vi "HC-Sr501.vi"() -> ()   [LabVIEW 2021]
uses:
  <vilib>/MakerHub/LINX/Public/Peripherals/Digital/Digital Read 1 Chan.vi
  <vilib>/MakerHub/LINX/Public/Peripherals/Digital/Digital Read N Chans.vi
  <vilib>/MakerHub/LINX/Private/Local IO/LinxDigitalRead.vi
  <vilib>/MakerHub/LINX/Public/Utilities/Check Channel.vi
  <vilib>/MakerHub/LINX/Public/Utilities/Open Serial.vi
  <vilib>/MakerHub/LINX/Public/Sensors/Motion/Servo/Servo Open One Channel.vi
  <vilib>/MakerHub/LINX/Private/Utilties/Generate Error.vi
  <vilib>/MakerHub/LINX/Public/Sensors/Motion/Servo/Servo Set Pulse Width One Channel.vi
  <vilib>/MakerHub/LINX/Public/Sensors/Motion/Servo/Servo Close One Channel.vi
  <vilib>/MakerHub/LINX/LMH-LINX.lvlib
  <vilib>/MakerHub/LINX/Public/Sensors/Motion/Servo/Servo.lvlib
panel:
  out "DOOR":bool
  in  "stop":bool
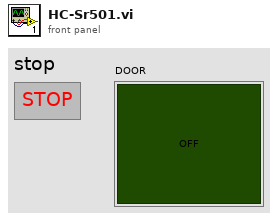
[diagram p1: front panel]
types:
  T1 = typedef "LMH-LINX.lvlib/LINX Ref.ctl" = cluster{"IO":T2, "Interface":T3, "LINX Device Config":T4}
  T2 = typedef "LMH-LINX.lvlib/Platform.ctl" = enum16{"Remote", "Local"}
  T3 = typedef "LMH-LINX.lvlib/Interface.ctl" = enum16{"Serial", "TCP"}
  T4 = typedef "LMH-LINX.lvlib/Device.lvlib/LINX Device Config.ctl" = cluster{"Interface":T3, "COM Port":refnum<visa-resource-name>, "TCP Configuration":T5, "Device Family":u8, "Device ID":u8, "Device Name":string, "TCP Ref":refnum<k5>, "Channels":T6}
  T5 = typedef "LMH-LINX.lvlib/Device.lvlib/TCP Config.ctl" = cluster{"IP Address":string, "Port":u16}
  T6 = typedef "LMH-LINX.lvlib/Channels.ctl" = cluster{"DI":u8[], "DO":u8[], "AI":u8[], "AO":u8[], "PWM":u8[], "QE":u8[], "UART":u8[], "I2C 2":u8[], "SPI":u8[], "CAN":u8[], "Servo":u8[], "AI Ref (V)":dbl, "AI Resolution (Bits)":u8, "AO Ref (V)":dbl, "AO Resolution (Bits)":u8}
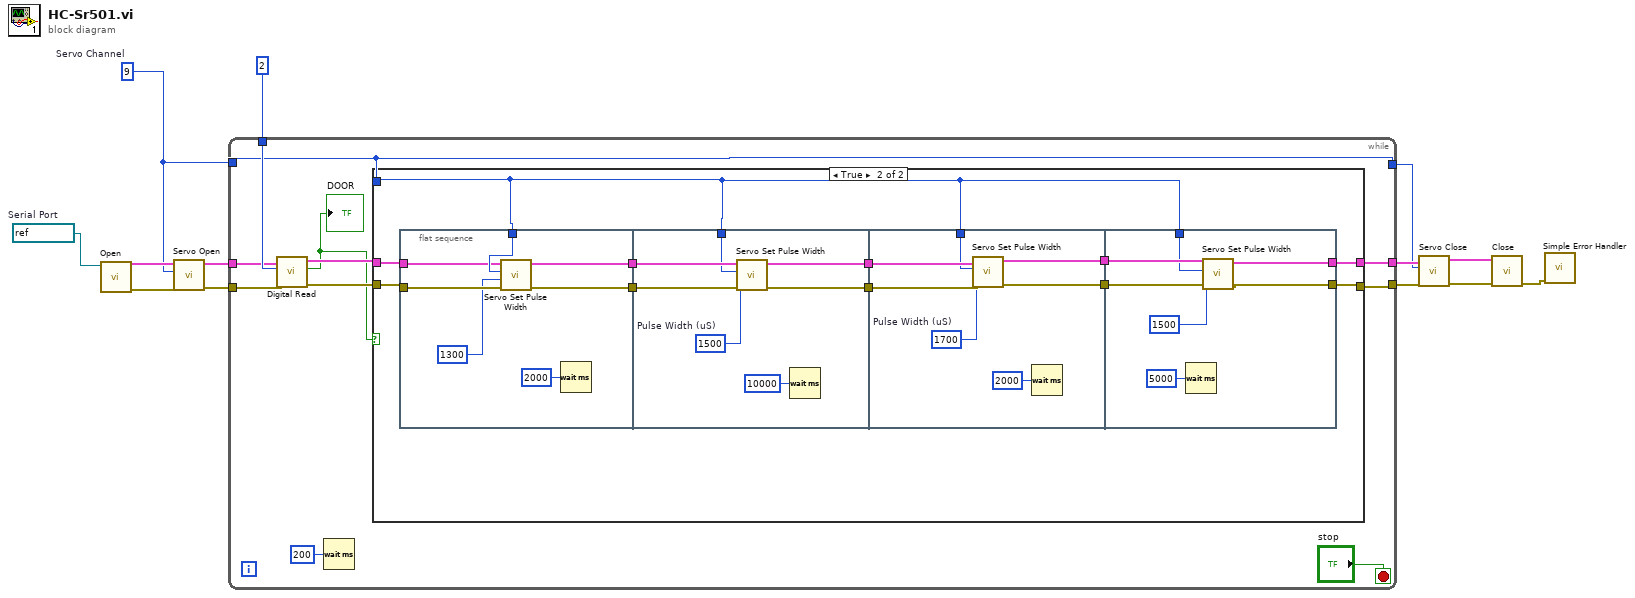
[diagram p0: block diagram]
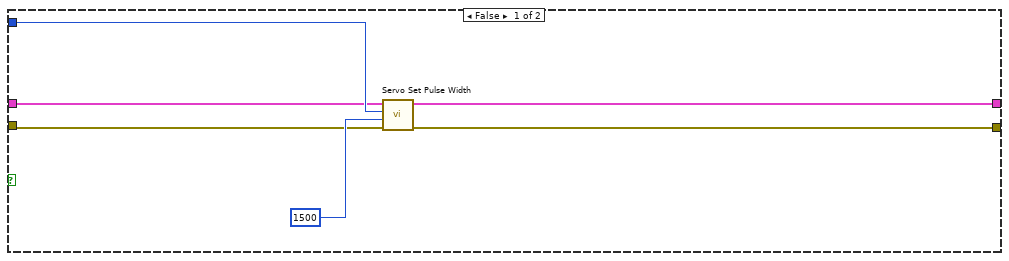
[diagram p2: hidden frame]
diagram:
  w11 = refnum<visa-resource-name> "COM3"  # Serial Port
  w7 = u8 9  # Servo Channel
  n1 = call-poly <vilib>:"Open.vi"("Serial Port"=w11) -> ("Error Out"=w12:errorcluster, "LINX Resource"=w13:T1)  [unwired: 8 in, 1 out]
  n2 = call-poly <vilib>:"Servo Open.vi"("Error In"=w12, "Servo Channel"=w7, "LINX Resource"=w13) -> ("Error Out"=w6:errorcluster, "LINX Resource"=w8:T1)  [unwired: 7 in]
  n3 = while {
    tunnel: [w15] -> w3
    tunnel: w8 -> [w17]
    tunnel: w7 -> [w15]
    tunnel: w6 -> [w16]
    tunnel: [w20] -> w5
    tunnel: [w21] -> w4
    tunnel: u8 2 ("DI Channel") -> [w18]
    stop <- "stop" stop-if-true
    n4 = call-poly <vilib>:"Digital Read.vi"("Error In"=w16, "DI Channel"=w18, "LINX Resource"=w17) -> ("Error Out"=w22:errorcluster, "DI Value"=w14:bool, "LINX Resource"=w19:T1)  [unwired: 6 in]
    "DOOR" <- w14
    n5 = Wait (ms)(milliseconds to wait=u32 200) -> ()  [unwired: 1 out]
    n6 = case shown="True" w14 {
      tunnel: w19 -> [w27 w34]
      tunnel: w22 -> [w28 w33]
      tunnel: [w26 w31] -> w21
      tunnel: [w25 w32] -> w20
      tunnel: w15 -> [w30 w41]
      frame False {
        n7 = call-poly <vilib>:"Servo Set Pulse Width.vi"("Error In"=w28, "Pulse Width (uS)"=u16 1500, "Servo Channel"=w30, "LINX Resource"=w27) -> ("Error Out"=w25:errorcluster, "LINX Resource"=w26:T1)  [unwired: 6 in]
      }
      frame True {
        n8 = flat-sequence {
          tunnel: [w48] -> w40
          tunnel: [w47] -> w39
          tunnel: w41 -> [w46]
          tunnel: w33 -> [w44]
          tunnel: w34 -> [w43]
          tunnel: w40 -> [w55]
          tunnel: [w54] -> w38
          tunnel: w39 -> [w53]
          tunnel: [w52] -> w37
          tunnel: w41 -> [w51]
          tunnel: w38 -> [w62]
          tunnel: [w61] -> w36
          tunnel: w37 -> [w60]
          tunnel: [w59] -> w35
          tunnel: w41 -> [w58]
          tunnel: w36 -> [w69]
          tunnel: [w68] -> w32
          tunnel: w35 -> [w67]
          tunnel: [w66] -> w31
          tunnel: w41 -> [w65]
          frame #0 {
            n9 = call-poly <vilib>:"Servo Set Pulse Width.vi"("Error In"=w44, "Pulse Width (uS)"=u16 1300, "Servo Channel"=w46, "LINX Resource"=w43) -> ("Error Out"=w48:errorcluster, "LINX Resource"=w47:T1)  [unwired: 6 in]
            n10 = Wait (ms)(milliseconds to wait=u32 2000) -> ()  [unwired: 1 out]
          }
          frame #1 {
            w50 = u16 1500  # Pulse Width (uS)
            n11 = call-poly <vilib>:"Servo Set Pulse Width.vi"("Error In"=w55, "Pulse Width (uS)"=w50, "Servo Channel"=w51, "LINX Resource"=w53) -> ("Error Out"=w54:errorcluster, "LINX Resource"=w52:T1)  [unwired: 6 in]
            n12 = Wait (ms)(milliseconds to wait=u32 10000) -> ()  [unwired: 1 out]
          }
          frame #2 {
            w57 = u16 1700  # Pulse Width (uS)
            n13 = call-poly <vilib>:"Servo Set Pulse Width.vi"("Error In"=w62, "Pulse Width (uS)"=w57, "Servo Channel"=w58, "LINX Resource"=w60) -> ("Error Out"=w61:errorcluster, "LINX Resource"=w59:T1)  [unwired: 6 in]
            n14 = Wait (ms)(milliseconds to wait=u32 2000) -> ()  [unwired: 1 out]
          }
          frame #3 {
            n15 = Wait (ms)(milliseconds to wait=u32 5000) -> ()  [unwired: 1 out]
            n16 = call-poly <vilib>:"Servo Set Pulse Width.vi"("Error In"=w69, "Pulse Width (uS)"=u16 1500, "Servo Channel"=w65, "LINX Resource"=w67) -> ("Error Out"=w68:errorcluster, "LINX Resource"=w66:T1)  [unwired: 6 in]
          }
        }
      }
    }
  }
  n17 = call-poly <vilib>:"Servo Close.vi"("Error In"=w5, "Servo Channel"=w3, "LINX Resource"=w4) -> ("Error Out"=w9:errorcluster, "LINX Resource"=w10:T1)  [unwired: 7 in]
  n18 = call <vilib>:"Close.vi"("Error In"=w9, "LINX Resource"=w10) -> ("Error Out"=w2:errorcluster)  [unwired: 9 in]
  n19 = call <vilib>:"Simple Error Handler.vi"("error in (no error)"=w2) -> ()  [unwired: 4 in, 5 out]
